vi "Load config.vi"(8 "error in":errorcluster, 10 "config file path":path, 11 "Config in":refnum<class "Config.lvclass">) -> (0 "error out":errorcluster, 3 "Config out":refnum<class "Config.lvclass">)   [LabVIEW 2026, in "TALOS.lvlib" / "Classes.lvlib" / "Config.lvclass"]
doc: "This VI loads config parameters from the specified file into a map in the private data of this class and it saves the file's path in private data. If the file path is empty, it uses the file path from private data (it can be used for reloading configurations after changing the content of the config file)."
uses:
  Config.lvclass
  Config.lvclass/Config.ctl
  <vilib>/Utility/config.llb/Read Key (String).vi
  <vilib>/Utility/config.llb/NI_LVConfig.lvlib
panel:
  out "section names":string[](array[string])
  out "key names":string[][](array[string])
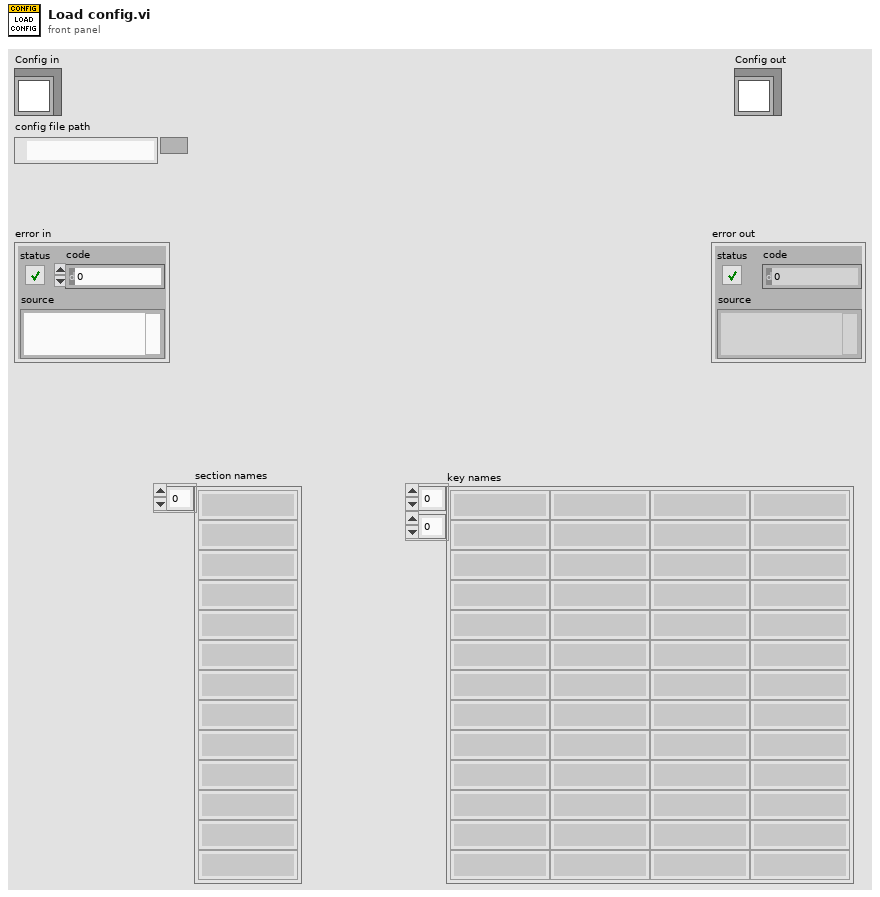
[diagram p1: front panel]
types:
  T1 = typedef "NI_LVConfig.lvlib/Config Data RefNum.ctl" = refnum<k1>
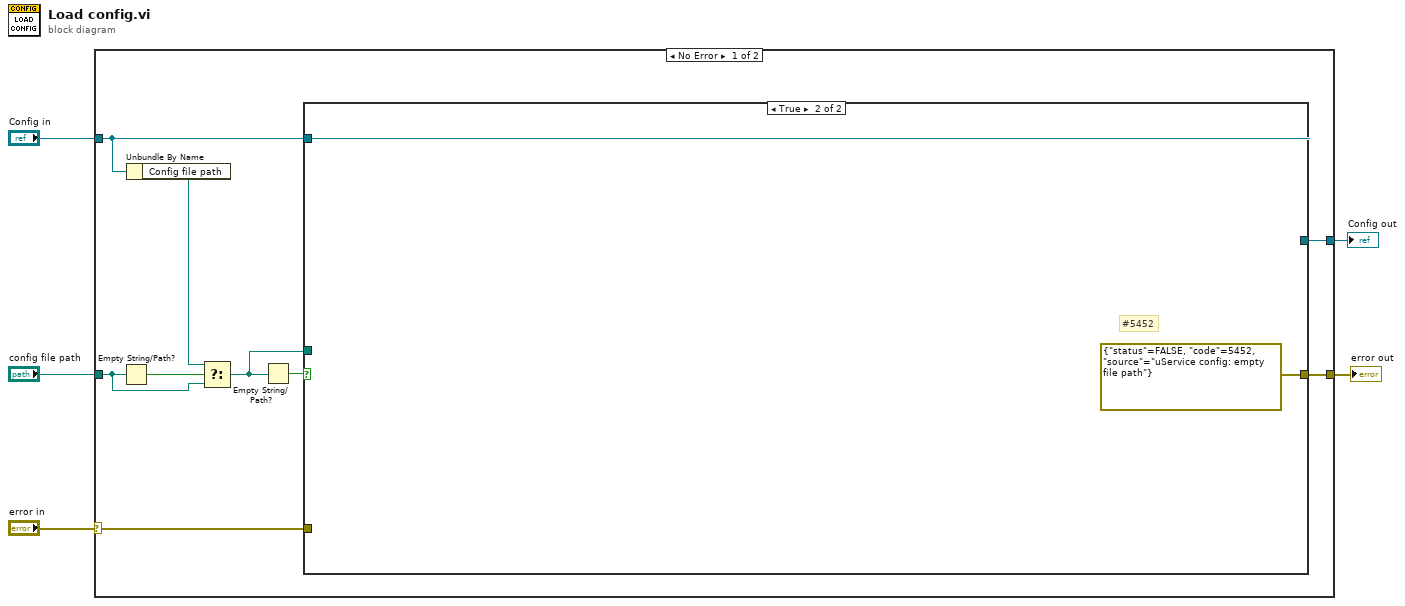
[diagram p0: block diagram]
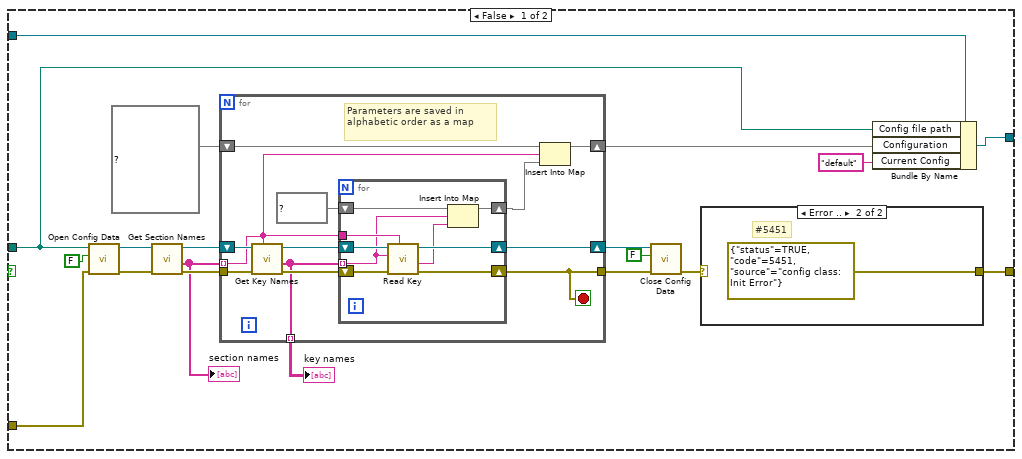
[diagram p2: hidden frame]
diagram:
  n1 = case shown="No Error" "error in" {
    selector: "error in" -> [w12 w60]
    tunnel: [w14 w60] -> w5
    tunnel: "config file path" -> [w9 _]
    tunnel: [w13 w59] -> w4
    tunnel: "Config in" -> [w11 w59]
    frame No Error {
      n2 = Empty String/Path?(string/path=w9) -> (empty?=w10:bool)
      n3 = Unbundle By Name(w11) -> ("Config file path"=w8:path)
      n4 = Select(t=w8, s=w10, f=w9) -> (s? t:f=w6:path)
      n5 = Empty String/Path?(string/path=w6) -> (empty?=w7:bool)
      n6 = case shown="True" w7 {
        tunnel: w6 -> [w31 _]
        tunnel: [w32 w57] -> w13
        tunnel: [w33 errorcluster {"status"=FALSE, "code"=5452, "source"="uService config: empty file path"} ("error IO")] -> w14
        tunnel: w11 -> [w30 w57]
        tunnel: w12 -> [w16 _]
        frame False {
          n7 = call <vilib>:"Open Config Data.vi"("error in (no error)"=w16, "create file if necessary (T)"=FALSE, "configuration file path"=w31) -> ("error out"=w28:errorcluster, "refnum"=w27:T1)  [unwired: 6 in, 1 out]
          n8 = call <vilib>:"Get Section Names.vi"("error in (no error)"=w28, "refnum"=w27) -> ("error out"=w25:errorcluster, "section names"=w24:string[], "refnum out"=w26:T1)  [unwired: 7 in]
          "section names" <- w24
          n9 = for {
            tunnel: w25 -> [w44]
            tunnel: w24 -> [w35] mode=indexing
            tunnel: [w37] -> w23 mode=indexing
            tunnel: [w38] -> w22
            shift-right: [w41] -> w17
            shift-left: map{string, map{string, string}} {} ("Configuration") -> [w40]
            shift-right: [w39] -> w21
            shift-left: w26 -> [w45]
            stop <- w38 stop-if-true
            # "Parameters are saved in alphabetic order as a map"
            n10 = call <vilib>:"Get Key Names.vi"("section"=w35, "error in (no error)"=w44, "refnum"=w45) -> ("error out"=w42:errorcluster, "key names"=w37:string[], "refnum out"=w43:T1)  [unwired: 5 in, 1 out]
            n11 = for {
              shift-right: [w52] -> w39
              shift-left: w43 -> [w54]
              shift-right: [w51] -> w38
              shift-left: w42 -> [w53]
              shift-right: [w48] -> w34
              shift-left: map{string, string} {} ("Size: 0") -> [w50]
              tunnel: w37 -> [w47] mode=indexing
              tunnel: w35 -> [w49]
              n12 = call-poly <vilib>:"Read Key.vi"("section"=w49, "error in (no error)"=w53, "key"=w47, "refnum"=w54) -> ("error out"=w51:errorcluster, "value"=w46:string, "refnum out"=w52:T1)  [unwired: 4 in, 1 out]
              n13 = Insert Into Map(map in=w50, key=w47, value=w46) -> (map out=w48:map{string, string})  [unwired: 2 out]
            }
            n14 = Insert Into Map(map in=w40, key=w35, value=w34) -> (map out=w41:map{string, map{string, string}})  [unwired: 2 out]
          }
          "key names" <- w23
          n15 = call <vilib>:"Close Config Data.vi"("error in (no error)"=w22, "write file if changed (T)"=FALSE, "refnum"=w21) -> ("error out"=w19:errorcluster)  [unwired: 7 in, 1 out]
          n16 = case shown="Error .." w19 {
            selector: w19 -> [w55 _]
            tunnel: [w55 errorcluster {"status"=TRUE, "code"=5451, "source"="config class: Init Error"} ("error IO")] -> w33
            frame No Error {
            }
            frame Error {
              # "#5451"
            }
          }
          n17 = Bundle By Name(cluster=w30, "Config file path"=w31, "Configuration"=w17, "Current Config"="default") -> (w32:refnum<class "Config.lvclass">)
        }
        frame True {
          # "#5452"
        }
      }
    }
    frame Error {
    }
  }
  "error out" <- w5
  "Config out" <- w4
